vi "IMAQ FPGA Configure Image Transfer to Target.vi"   [LabVIEW 2017, in "NI_VDM_FPGA_Basics.lvlib"]
doc: "Configures the transfer of an image from the host processor to the target FPGA via a DMA FIFO. If the <B>Image Size</B> control specifies non-zero <B>Width</B> and <B>Height</B> values, then the image referenced by <B>Image</B> will be resized to match those values. Otherwise, the original image size is preserved. The resulting image size will be set to the FPGA VI front panel control that matches the IMAQ FPGA Image Size.ctl typedef. In addition, a reference will be opened to the DMA FIFO that will be used to transfer the image from the host computer to the target FPGA."
uses:
  <vilib>/visionFPGA/NI_VDM_FPGA_Basics.lvlib
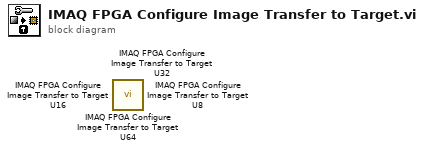
[diagram p0: block diagram]
diagram:
  n1 = call <vilib>:"IMAQ FPGA Configure Image Transfer to Target U64.vi"() -> ()  [unwired: 8 in, 4 out]
  n2 = call <vilib>:"IMAQ FPGA Configure Image Transfer to Target U32.vi"() -> ()  [unwired: 8 in, 4 out]
  n3 = call <vilib>:"IMAQ FPGA Configure Image Transfer to Target U16.vi"() -> ()  [unwired: 8 in, 4 out]
  n4 = call <vilib>:"IMAQ FPGA Configure Image Transfer to Target U8.vi"() -> ()  [unwired: 8 in, 4 out]
